vi "offsets_R-W.vi"(1 "Offset_R/W":bool, 2 "parameter":string="Offset_Group1", 3 "Real IMon":dbl[](array[numeric])=[0.0, 0.0, 0.0, 0.0, 0.0, 0.0, 0.0, 0.0, 0.0, 0.0, 0.0, 0.0] format="%.3f") -> (0 "corection IMon":dbl[](array[numeric]) format="%.3f")   [LabVIEW 2018]
uses:
  <vilib>/Utility/config.llb/Read Key (Double).vi
  <vilib>/Utility/config.llb/Write Key (Double).vi
  <vilib>/Utility/config.llb/NI_LVConfig.lvlib
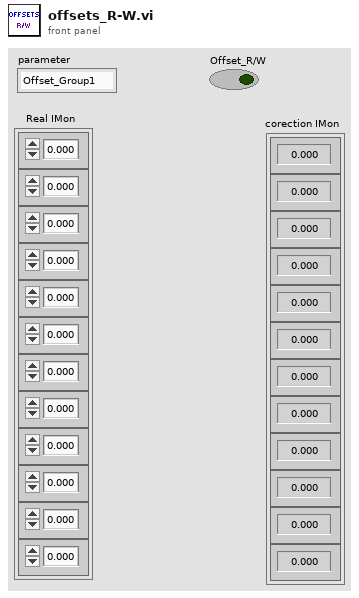
[diagram p1: front panel]
types:
  T1 = typedef "NI_LVConfig.lvlib/Config Data RefNum.ctl" = refnum<k1>
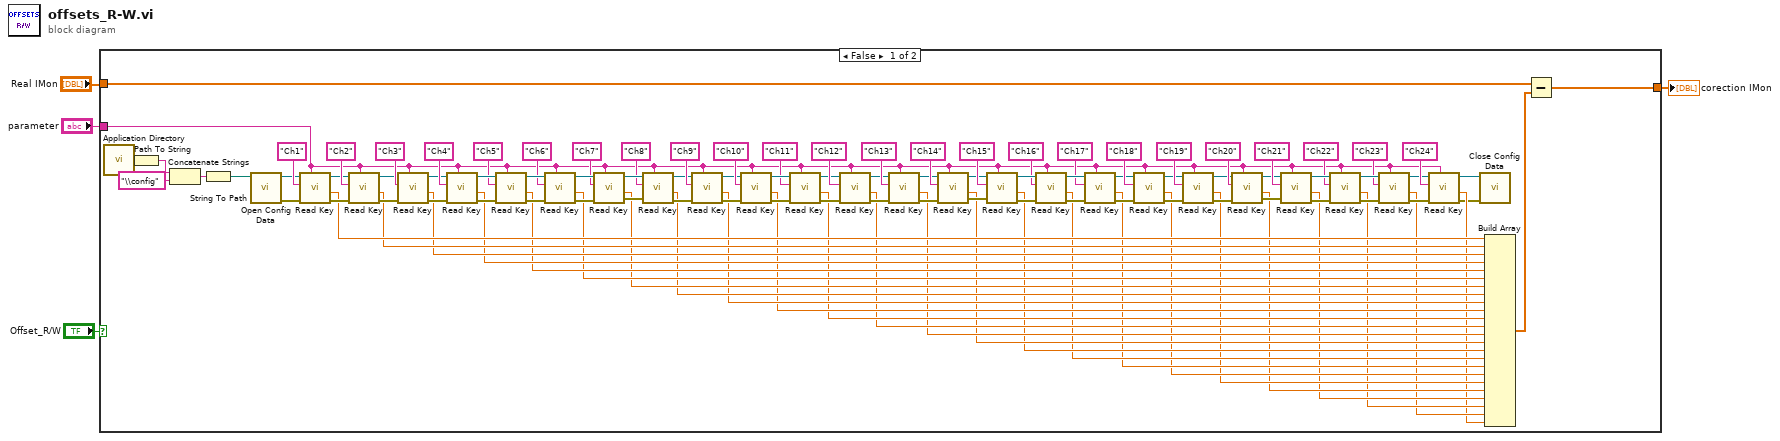
[diagram p0: block diagram]
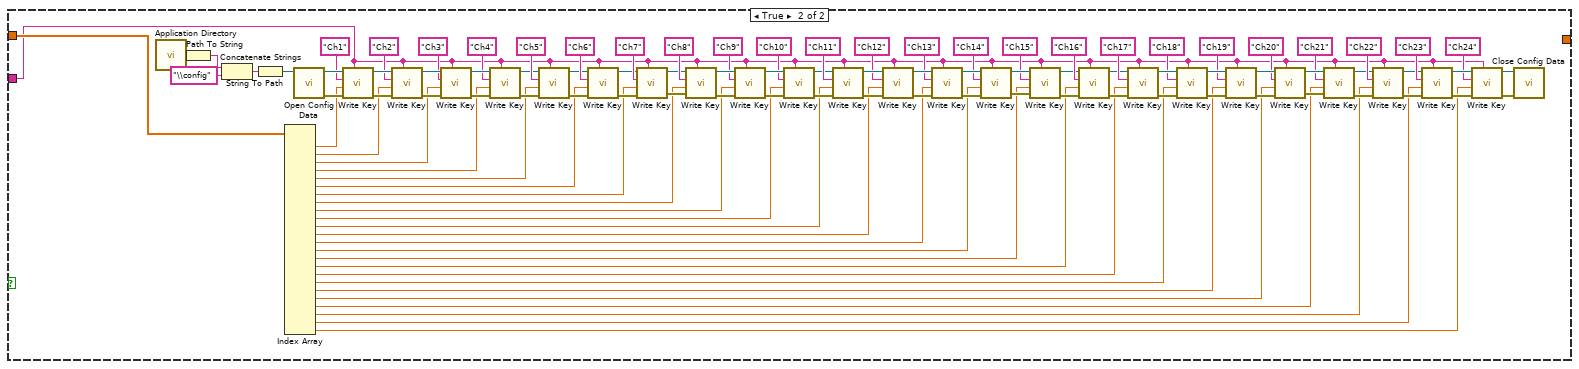
[diagram p2: hidden frame]
diagram:
  n1 = case shown="False" "Offset_R/W" {
    tunnel: "Real IMon" -> [w9 w117]
    tunnel: [w8 _] -> w2
    tunnel: "parameter" -> [w5 w112]
    frame False {
      n2 = call <vilib>:"Application Directory.vi"() -> ("Application Directory"=w12:path)
      n3 = Path To String(path=w12) -> (string=w13:string)
      n4 = Concatenate Strings(w13, "\\config" ("string")) -> (w15:string)
      n5 = String To Path(string=w15) -> (path=w11:path)
      n6 = call <vilib>:"Open Config Data.vi"("configuration file path"=w11) -> ("error out"=w49:errorcluster, "refnum"=w50:T1)  [unwired: 8 in, 1 out]
      n7 = call-poly <vilib>:"Read Key.vi"("section"=w5, "error in (no error)"=w49, "key"="Ch1", "refnum"=w50) -> ("error out"=w46:errorcluster, "value"=w39:dbl, "refnum out"=w47:T1)  [unwired: 4 in, 1 out]
      n8 = call-poly <vilib>:"Read Key.vi"("section"=w5, "error in (no error)"=w46, "key"="Ch2", "refnum"=w47) -> ("error out"=w43:errorcluster, "value"=w38:dbl, "refnum out"=w44:T1)  [unwired: 4 in, 1 out]
      n9 = call-poly <vilib>:"Read Key.vi"("section"=w5, "error in (no error)"=w43, "key"="Ch3", "refnum"=w44) -> ("error out"=w40:errorcluster, "value"=w37:dbl, "refnum out"=w41:T1)  [unwired: 4 in, 1 out]
      n10 = call-poly <vilib>:"Read Key.vi"("section"=w5, "error in (no error)"=w40, "key"="Ch4", "refnum"=w41) -> ("error out"=w63:errorcluster, "value"=w36:dbl, "refnum out"=w62:T1)  [unwired: 4 in, 1 out]
      n11 = call-poly <vilib>:"Read Key.vi"("section"=w5, "error in (no error)"=w63, "key"="Ch5", "refnum"=w62) -> ("error out"=w55:errorcluster, "value"=w35:dbl, "refnum out"=w54:T1)  [unwired: 4 in, 1 out]
      n12 = call-poly <vilib>:"Read Key.vi"("section"=w5, "error in (no error)"=w55, "key"="Ch6", "refnum"=w54) -> ("error out"=w58:errorcluster, "value"=w34:dbl, "refnum out"=w57:T1)  [unwired: 4 in, 1 out]
      n13 = call-poly <vilib>:"Read Key.vi"("section"=w5, "error in (no error)"=w58, "key"="Ch7", "refnum"=w57) -> ("error out"=w61:errorcluster, "value"=w33:dbl, "refnum out"=w60:T1)  [unwired: 4 in, 1 out]
      n14 = call-poly <vilib>:"Read Key.vi"("section"=w5, "error in (no error)"=w61, "key"="Ch8", "refnum"=w60) -> ("error out"=w79:errorcluster, "value"=w32:dbl, "refnum out"=w80:T1)  [unwired: 4 in, 1 out]
      n15 = call-poly <vilib>:"Read Key.vi"("section"=w5, "error in (no error)"=w79, "key"="Ch9", "refnum"=w80) -> ("error out"=w75:errorcluster, "value"=w31:dbl, "refnum out"=w74:T1)  [unwired: 4 in, 1 out]
      n16 = call-poly <vilib>:"Read Key.vi"("section"=w5, "error in (no error)"=w75, "key"="Ch10", "refnum"=w74) -> ("error out"=w78:errorcluster, "value"=w30:dbl, "refnum out"=w77:T1)  [unwired: 4 in, 1 out]
      n17 = call-poly <vilib>:"Read Key.vi"("section"=w5, "error in (no error)"=w78, "key"="Ch11", "refnum"=w77) -> ("error out"=w64:errorcluster, "value"=w29:dbl, "refnum out"=w65:T1)  [unwired: 4 in, 1 out]
      n18 = call-poly <vilib>:"Read Key.vi"("section"=w5, "error in (no error)"=w64, "key"="Ch12", "refnum"=w65) -> ("error out"=w71:errorcluster, "value"=w28:dbl, "refnum out"=w72:T1)  [unwired: 4 in, 1 out]
      n19 = call-poly <vilib>:"Read Key.vi"("section"=w5, "error in (no error)"=w71, "key"="Ch13", "refnum"=w72) -> ("error out"=w69:errorcluster, "value"=w27:dbl, "refnum out"=w70:T1)  [unwired: 4 in, 1 out]
      n20 = call-poly <vilib>:"Read Key.vi"("section"=w5, "error in (no error)"=w69, "key"="Ch14", "refnum"=w70) -> ("error out"=w66:errorcluster, "value"=w26:dbl, "refnum out"=w67:T1)  [unwired: 4 in, 1 out]
      n21 = call-poly <vilib>:"Read Key.vi"("section"=w5, "error in (no error)"=w66, "key"="Ch15", "refnum"=w67) -> ("error out"=w111:errorcluster, "value"=w25:dbl, "refnum out"=w110:T1)  [unwired: 4 in, 1 out]
      n22 = call-poly <vilib>:"Read Key.vi"("section"=w5, "error in (no error)"=w111, "key"="Ch16", "refnum"=w110) -> ("error out"=w109:errorcluster, "value"=w24:dbl, "refnum out"=w108:T1)  [unwired: 4 in, 1 out]
      n23 = call-poly <vilib>:"Read Key.vi"("section"=w5, "error in (no error)"=w109, "key"="Ch17", "refnum"=w108) -> ("error out"=w94:errorcluster, "value"=w23:dbl, "refnum out"=w95:T1)  [unwired: 4 in, 1 out]
      n24 = call-poly <vilib>:"Read Key.vi"("section"=w5, "error in (no error)"=w94, "key"="Ch18", "refnum"=w95) -> ("error out"=w102:errorcluster, "value"=w22:dbl, "refnum out"=w103:T1)  [unwired: 4 in, 1 out]
      n25 = call-poly <vilib>:"Read Key.vi"("section"=w5, "error in (no error)"=w102, "key"="Ch19", "refnum"=w103) -> ("error out"=w99:errorcluster, "value"=w21:dbl, "refnum out"=w100:T1)  [unwired: 4 in, 1 out]
      n26 = call-poly <vilib>:"Read Key.vi"("section"=w5, "error in (no error)"=w99, "key"="Ch20", "refnum"=w100) -> ("error out"=w96:errorcluster, "value"=w20:dbl, "refnum out"=w97:T1)  [unwired: 4 in, 1 out]
      n27 = call-poly <vilib>:"Read Key.vi"("section"=w5, "error in (no error)"=w96, "key"="Ch21", "refnum"=w97) -> ("error out"=w88:errorcluster, "value"=w19:dbl, "refnum out"=w87:T1)  [unwired: 4 in, 1 out]
      n28 = call-poly <vilib>:"Read Key.vi"("section"=w5, "error in (no error)"=w88, "key"="Ch22", "refnum"=w87) -> ("error out"=w92:errorcluster, "value"=w18:dbl, "refnum out"=w93:T1)  [unwired: 4 in, 1 out]
      n29 = call-poly <vilib>:"Read Key.vi"("section"=w5, "error in (no error)"=w92, "key"="Ch23", "refnum"=w93) -> ("error out"=w89:errorcluster, "value"=w17:dbl, "refnum out"=w90:T1)  [unwired: 4 in, 1 out]
      n30 = call-poly <vilib>:"Read Key.vi"("section"=w5, "error in (no error)"=w89, "key"="Ch24", "refnum"=w90) -> ("error out"=w6:errorcluster, "value"=w16:dbl, "refnum out"=w7:T1)  [unwired: 4 in, 1 out]
      n31 = call <vilib>:"Close Config Data.vi"("error in (no error)"=w6, "refnum"=w7) -> ()  [unwired: 8 in, 2 out]
      n32 = Build Array(w39, w38, w37, w36, w35, w34, w33, w32, w31, w30, w29, w28, w27, w26, w25, w24, w23, w22, w21, w20, w19, w18, w17, w16) -> (w10:dbl[])
      n33 = Subtract(x=w9, y=w10) -> (x-y=w8:dbl[])
    }
    frame True {
      n34 = call <vilib>:"Application Directory.vi"() -> ("Application Directory"=w118:path)
      n35 = Path To String(path=w118) -> (string=w119:string)
      n36 = Concatenate Strings(w119, "\\config" ("string")) -> (w115:string)
      n37 = String To Path(string=w115) -> (path=w116:path)
      n38 = Index Array(array=w117) -> (element #1=w144:dbl, element #2=w143:dbl, element #3=w142:dbl, element #4=w141:dbl, element #5=w140:dbl, element #6=w139:dbl, element #7=w138:dbl, element #8=w137:dbl, element #9=w136:dbl, element #10=w135:dbl, element #11=w134:dbl, element #12=w133:dbl, element #13=w132:dbl, element #14=w131:dbl, element #15=w130:dbl, element #16=w129:dbl, element #17=w128:dbl, element #18=w127:dbl, element #19=w126:dbl, element #20=w125:dbl, element #21=w124:dbl, element #22=w123:dbl, element #23=w122:dbl, element #24=w121:dbl)  [unwired: 24 in]
      n39 = call <vilib>:"Open Config Data.vi"("configuration file path"=w116) -> ("error out"=w207:errorcluster, "refnum"=w206:T1)  [unwired: 8 in, 1 out]
      n40 = call-poly <vilib>:"Write Key.vi"("section"=w112, "error in (no error)"=w207, "value"=w144, "key"="Ch1", "refnum"=w206) -> ("error out"=w210:errorcluster, "refnum out"=w209:T1)  [unwired: 4 in, 1 out]
      n41 = call-poly <vilib>:"Write Key.vi"("section"=w112, "error in (no error)"=w210, "value"=w143, "key"="Ch2", "refnum"=w209) -> ("error out"=w213:errorcluster, "refnum out"=w212:T1)  [unwired: 4 in, 1 out]
      n42 = call-poly <vilib>:"Write Key.vi"("section"=w112, "error in (no error)"=w213, "value"=w142, "key"="Ch3", "refnum"=w212) -> ("error out"=w216:errorcluster, "refnum out"=w215:T1)  [unwired: 4 in, 1 out]
      n43 = call-poly <vilib>:"Write Key.vi"("section"=w112, "error in (no error)"=w216, "value"=w141, "key"="Ch4", "refnum"=w215) -> ("error out"=w193:errorcluster, "refnum out"=w194:T1)  [unwired: 4 in, 1 out]
      n44 = call-poly <vilib>:"Write Key.vi"("section"=w112, "error in (no error)"=w193, "value"=w140, "key"="Ch5", "refnum"=w194) -> ("error out"=w201:errorcluster, "refnum out"=w202:T1)  [unwired: 4 in, 1 out]
      n45 = call-poly <vilib>:"Write Key.vi"("section"=w112, "error in (no error)"=w201, "value"=w139, "key"="Ch6", "refnum"=w202) -> ("error out"=w198:errorcluster, "refnum out"=w199:T1)  [unwired: 4 in, 1 out]
      n46 = call-poly <vilib>:"Write Key.vi"("section"=w112, "error in (no error)"=w198, "value"=w138, "key"="Ch7", "refnum"=w199) -> ("error out"=w195:errorcluster, "refnum out"=w196:T1)  [unwired: 4 in, 1 out]
      n47 = call-poly <vilib>:"Write Key.vi"("section"=w112, "error in (no error)"=w195, "value"=w137, "key"="Ch8", "refnum"=w196) -> ("error out"=w177:errorcluster, "refnum out"=w176:T1)  [unwired: 4 in, 1 out]
      n48 = call-poly <vilib>:"Write Key.vi"("section"=w112, "error in (no error)"=w177, "value"=w136, "key"="Ch9", "refnum"=w176) -> ("error out"=w181:errorcluster, "refnum out"=w182:T1)  [unwired: 4 in, 1 out]
      n49 = call-poly <vilib>:"Write Key.vi"("section"=w112, "error in (no error)"=w181, "value"=w135, "key"="Ch10", "refnum"=w182) -> ("error out"=w178:errorcluster, "refnum out"=w179:T1)  [unwired: 4 in, 1 out]
      n50 = call-poly <vilib>:"Write Key.vi"("section"=w112, "error in (no error)"=w178, "value"=w134, "key"="Ch11", "refnum"=w179) -> ("error out"=w192:errorcluster, "refnum out"=w191:T1)  [unwired: 4 in, 1 out]
      n51 = call-poly <vilib>:"Write Key.vi"("section"=w112, "error in (no error)"=w192, "value"=w133, "key"="Ch12", "refnum"=w191) -> ("error out"=w185:errorcluster, "refnum out"=w184:T1)  [unwired: 4 in, 1 out]
      n52 = call-poly <vilib>:"Write Key.vi"("section"=w112, "error in (no error)"=w185, "value"=w132, "key"="Ch13", "refnum"=w184) -> ("error out"=w187:errorcluster, "refnum out"=w186:T1)  [unwired: 4 in, 1 out]
      n53 = call-poly <vilib>:"Write Key.vi"("section"=w112, "error in (no error)"=w187, "value"=w131, "key"="Ch14", "refnum"=w186) -> ("error out"=w190:errorcluster, "refnum out"=w189:T1)  [unwired: 4 in, 1 out]
      n54 = call-poly <vilib>:"Write Key.vi"("section"=w112, "error in (no error)"=w190, "value"=w130, "key"="Ch15", "refnum"=w189) -> ("error out"=w145:errorcluster, "refnum out"=w146:T1)  [unwired: 4 in, 1 out]
      n55 = call-poly <vilib>:"Write Key.vi"("section"=w112, "error in (no error)"=w145, "value"=w129, "key"="Ch16", "refnum"=w146) -> ("error out"=w147:errorcluster, "refnum out"=w148:T1)  [unwired: 4 in, 1 out]
      n56 = call-poly <vilib>:"Write Key.vi"("section"=w112, "error in (no error)"=w147, "value"=w128, "key"="Ch17", "refnum"=w148) -> ("error out"=w162:errorcluster, "refnum out"=w161:T1)  [unwired: 4 in, 1 out]
      n57 = call-poly <vilib>:"Write Key.vi"("section"=w112, "error in (no error)"=w162, "value"=w127, "key"="Ch18", "refnum"=w161) -> ("error out"=w154:errorcluster, "refnum out"=w153:T1)  [unwired: 4 in, 1 out]
      n58 = call-poly <vilib>:"Write Key.vi"("section"=w112, "error in (no error)"=w154, "value"=w126, "key"="Ch19", "refnum"=w153) -> ("error out"=w157:errorcluster, "refnum out"=w156:T1)  [unwired: 4 in, 1 out]
      n59 = call-poly <vilib>:"Write Key.vi"("section"=w112, "error in (no error)"=w157, "value"=w125, "key"="Ch20", "refnum"=w156) -> ("error out"=w160:errorcluster, "refnum out"=w159:T1)  [unwired: 4 in, 1 out]
      n60 = call-poly <vilib>:"Write Key.vi"("section"=w112, "error in (no error)"=w160, "value"=w124, "key"="Ch21", "refnum"=w159) -> ("error out"=w168:errorcluster, "refnum out"=w169:T1)  [unwired: 4 in, 1 out]
      n61 = call-poly <vilib>:"Write Key.vi"("section"=w112, "error in (no error)"=w168, "value"=w123, "key"="Ch22", "refnum"=w169) -> ("error out"=w164:errorcluster, "refnum out"=w163:T1)  [unwired: 4 in, 1 out]
      n62 = call-poly <vilib>:"Write Key.vi"("section"=w112, "error in (no error)"=w164, "value"=w122, "key"="Ch23", "refnum"=w163) -> ("error out"=w167:errorcluster, "refnum out"=w166:T1)  [unwired: 4 in, 1 out]
      n63 = call-poly <vilib>:"Write Key.vi"("section"=w112, "error in (no error)"=w167, "value"=w121, "key"="Ch24", "refnum"=w166) -> ("error out"=w113:errorcluster, "refnum out"=w114:T1)  [unwired: 4 in, 1 out]
      n64 = call <vilib>:"Close Config Data.vi"("error in (no error)"=w113, "refnum"=w114) -> ()  [unwired: 8 in, 2 out]
    }
  }
  "corection IMon" <- w2
